vi "Digital Gain (Pre).vi"(0 "data in":T1[](array[typedef])=[{"I"=0.0, "Q"=0.0, "overflow"=FALSE}, {"I"=0.0, "Q"=0.0, "overflow"=FALSE}], 9 "input valid":bool, 11 "gen in":refnum<class "niUSRP Tx DSP v2 FPGA.lvclass">, 12 "ready for output (T)":bool=TRUE) -> (4 "data out":T1[](array[typedef]), 10 "output valid":bool, 14 "ready for input":bool, 15 "gen out":refnum<class "niUSRP Tx DSP v2 FPGA.lvclass">)   [LabVIEW 2025, in "niUSRP Tx DSP v2 FPGA.lvclass"]
uses:
  niUSRP Tx DSP v2 FPGA.lvclass
  <instrlib>/_niInstr/DSP/v1/Shared/Public/IQ Data.ctl
  <instrlib>/_niInstr/DSP Control/Interface/v1/FPGA/Digital Gain/IQ 18-bit/Digital Gain Interface (IQ 18-bit).lvclass
  <instrlib>/_niInstr/Basic Elements/v1/FPGA/niInstr Basic Elements v1 FPGA.lvlib
  <instrlib>/_niInstr/DSP/v1/Shared/niInstr DSP v1 Shared.lvlib
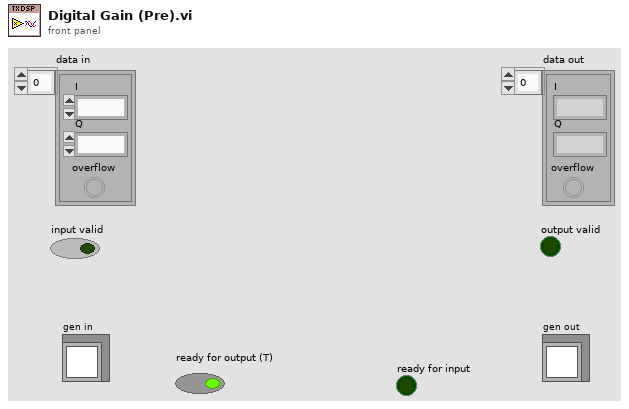
[diagram p1: front panel]
types:
  T1 = typedef "niInstr DSP v1 Shared.lvlib/IQ Data.ctl" = cluster{"I":fxp<+/-,18,1>, "Q":fxp<+/-,18,1>, "overflow":bool}
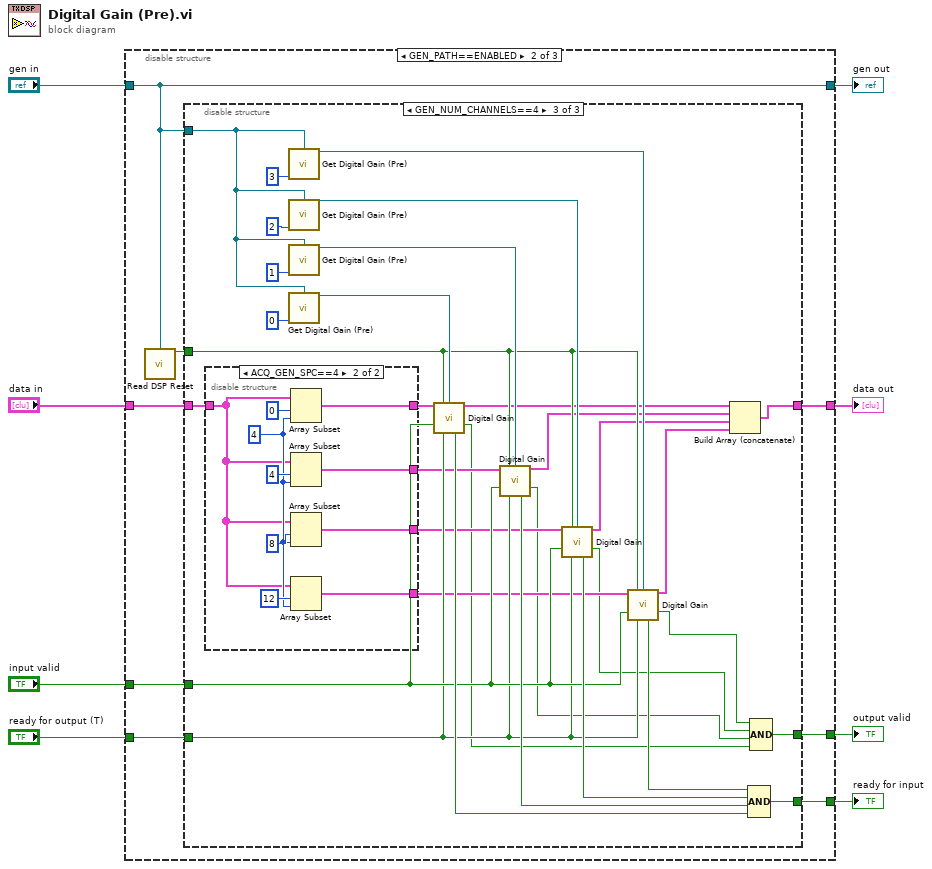
[diagram p0: block diagram]
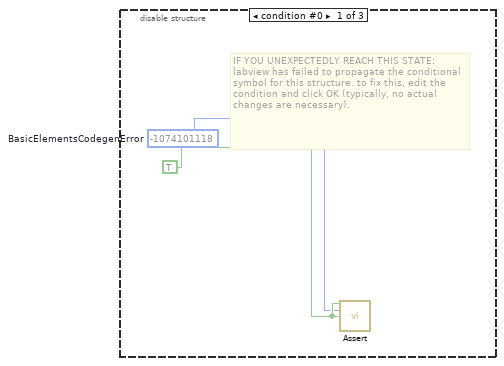
[diagram p2: hidden frame]
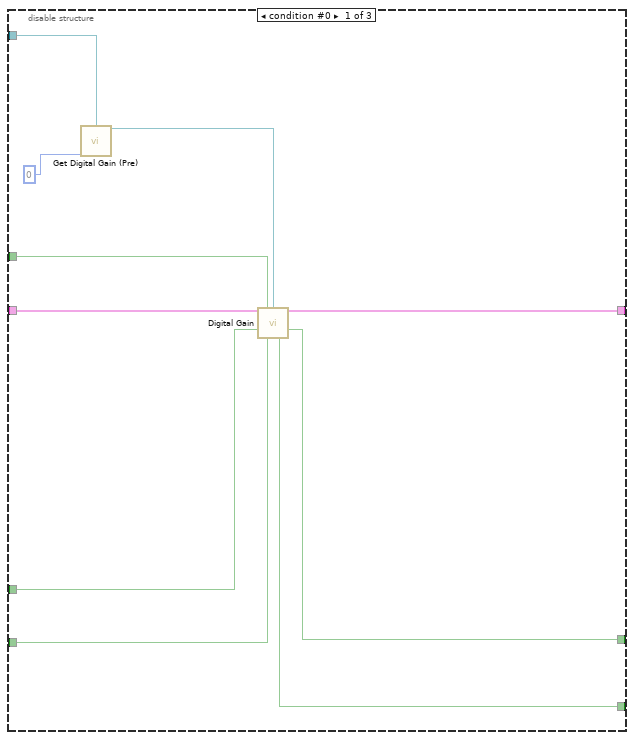
[diagram p3: hidden frame]
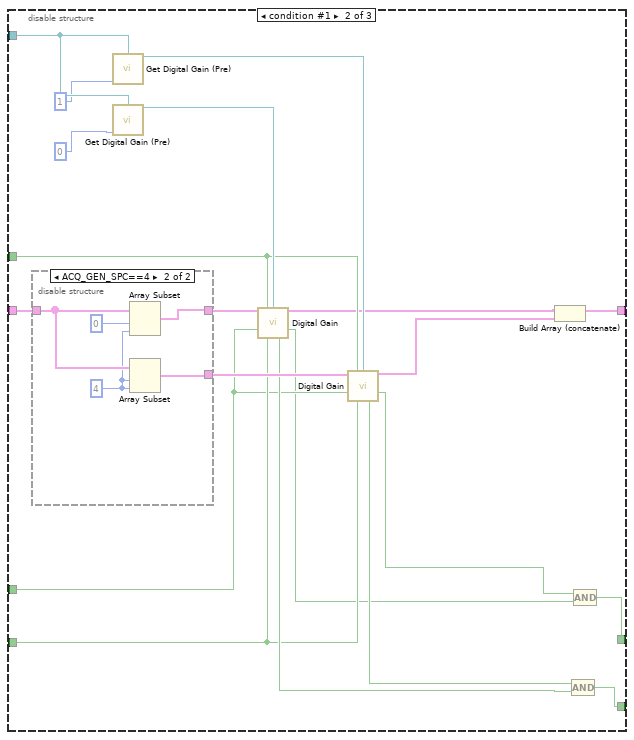
[diagram p4: hidden frame]
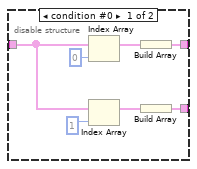
[diagram p5: hidden frame]
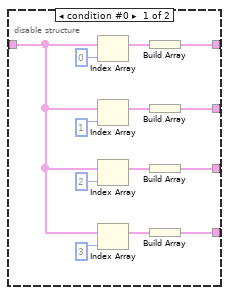
[diagram p6: hidden frame]
diagram:
  n1 = disable-structure shown="GEN_PATH==ENABLED" {
    disable-tunnel: [_ w18 w119] -> w8
    disable-tunnel: "input valid" -> [_ w17 w118]
    disable-tunnel: "ready for output (T)" -> [_ w16 w117]
    disable-tunnel: [_ w15 w118] -> w5
    disable-tunnel: "data in" -> [_ w14 w119]
    disable-tunnel: [_ w13 w117] -> w2
    disable-tunnel: "gen in" -> [_ w11 w116]
    disable-tunnel: [_ w11 w116] -> w1
    frame condition #0 {
      w10 = TRUE ("assert")
      w9 = -1074101118  # BasicElementsCodegenError
      # "IF YOU UNEXPECTEDLY REACH THIS STATE:\nlabview has failed to propagate the conditional symbol for this structure. to fix this, edit the condition and click OK (typically, no actual changes are necessary)."
      n2 = call <instrlib>:"Assert.vi"("assert"=w10, "error code"=w9, "enable show error"=w10) -> ()  [unwired: 13 in]
    }
    frame condition #1 (active) {
      n3 = call-dynamic "Read DSP Reset.vi"("gen"=w11) -> ("dsp reset"=w12:bool)  [unwired: 14 in]
      n4 = disable-structure shown="GEN_NUM_CHANNELS==4" {
        disable-tunnel: [w28 w42 w92] -> w18
        disable-tunnel: w17 -> [w27 w36 w75]
        disable-tunnel: w16 -> [w26 w37 w74]
        disable-tunnel: [w25 w41 w91] -> w15
        disable-tunnel: w14 -> [w24 w46 w73]
        disable-tunnel: [w23 w39 w89] -> w13
        disable-tunnel: w12 -> [w22 w33 w76]
        disable-tunnel: w11 -> [w20 w47 w83]
        frame condition #0 {
          n5 = call-dynamic "Get Digital Gain (Pre).vi"("gen"=w20, "ch"=u8 0) -> ("digital gain"=w21:refnum<class "Digital Gain Interface (IQ 18-bit).lvclass">)  [unwired: 13 in]
          n6 = call-dynamic "Digital Gain.vi"("data in"=w24, "reset"=w22, "digital gain"=w21, "input valid"=w27, "ready for output (T)"=w26) -> ("data out"=w28:T1[], "output valid"=w25:bool, "ready for input"=w23:bool)  [unwired: 7 in, 1 out]
        }
        frame condition #1 {
          n7 = disable-structure shown="ACQ_GEN_SPC==4" {
            disable-tunnel: w46 -> [w51 w58]
            disable-tunnel: [w50 w59] -> w45
            disable-tunnel: [w49 w57] -> w44
            frame condition #0 {
              n8 = Index Array(array=w51, index=0) -> (element=w55:T1)
              n9 = Index Array(array=w51, index=1) -> (element=w53:T1)
              n10 = Build Array(w55) -> (w50:T1[])
              n11 = Build Array(w53) -> (w49:T1[])
            }
            frame condition #1 (active) {
              w56 = 4 ("length")
              n12 = Array Subset(array=w58, index=0, length=w56) -> (w59:T1[])
              n13 = Array Subset(array=w58, index=w56, length=w56) -> (w57:T1[])
            }
          }
          n14 = call-dynamic "Get Digital Gain (Pre).vi"("gen"=w47, "ch"=u8 1) -> ("digital gain"=w43:refnum<class "Digital Gain Interface (IQ 18-bit).lvclass">)  [unwired: 13 in]
          n15 = call-dynamic "Get Digital Gain (Pre).vi"("gen"=w47, "ch"=u8 0) -> ("digital gain"=w48:refnum<class "Digital Gain Interface (IQ 18-bit).lvclass">)  [unwired: 13 in]
          n16 = call-dynamic "Digital Gain.vi"("data in"=w45, "reset"=w33, "digital gain"=w48, "input valid"=w36, "ready for output (T)"=w37) -> ("data out"=w32:T1[], "output valid"=w29:bool, "ready for input"=w40:bool)  [unwired: 7 in, 1 out]
          n17 = call-dynamic "Digital Gain.vi"("data in"=w44, "reset"=w33, "digital gain"=w43, "input valid"=w36, "ready for output (T)"=w37) -> ("data out"=w31:T1[], "output valid"=w30:bool, "ready for input"=w38:bool)  [unwired: 7 in, 1 out]
          n18 = Build Array (concatenate)(w32, w31) -> (w42:T1[])
          n19 = Compound Arithmetic op=AND(w38, w40) -> (w39:bool)
          n20 = Compound Arithmetic op=AND(w30, w29) -> (w41:bool)
        }
        frame condition #2 (active) {
          n21 = disable-structure shown="ACQ_GEN_SPC==4" {
            disable-tunnel: [w101 w109] -> w72
            disable-tunnel: [w100 w108] -> w71
            disable-tunnel: [w99 w107] -> w70
            disable-tunnel: w73 -> [w94 w110]
            disable-tunnel: [w93 w106] -> w69
            frame condition #0 {
              n22 = Index Array(array=w94, index=0) -> (element=w105:T1)
              n23 = Index Array(array=w94, index=1) -> (element=w103:T1)
              n24 = Index Array(array=w94, index=2) -> (element=w95:T1)
              n25 = Index Array(array=w94, index=3) -> (element=w97:T1)
              n26 = Build Array(w105) -> (w101:T1[])
              n27 = Build Array(w103) -> (w100:T1[])
              n28 = Build Array(w95) -> (w99:T1[])
              n29 = Build Array(w97) -> (w93:T1[])
            }
            frame condition #1 (active) {
              w111 = 4 ("length")
              n30 = Array Subset(array=w110, index=0, length=w111) -> (w109:T1[])
              n31 = Array Subset(array=w110, index=4, length=w111) -> (w108:T1[])
              n32 = Array Subset(array=w110, index=8, length=w111) -> (w107:T1[])
              n33 = Array Subset(array=w110, index=12, length=w111) -> (w106:T1[])
            }
          }
          n34 = call-dynamic "Get Digital Gain (Pre).vi"("gen"=w83, "ch"=u8 3) -> ("digital gain"=w77:refnum<class "Digital Gain Interface (IQ 18-bit).lvclass">)  [unwired: 13 in]
          n35 = call-dynamic "Get Digital Gain (Pre).vi"("gen"=w83, "ch"=u8 2) -> ("digital gain"=w78:refnum<class "Digital Gain Interface (IQ 18-bit).lvclass">)  [unwired: 13 in]
          n36 = call-dynamic "Get Digital Gain (Pre).vi"("gen"=w83, "ch"=u8 1) -> ("digital gain"=w81:refnum<class "Digital Gain Interface (IQ 18-bit).lvclass">)  [unwired: 13 in]
          n37 = call-dynamic "Get Digital Gain (Pre).vi"("gen"=w83, "ch"=u8 0) -> ("digital gain"=w82:refnum<class "Digital Gain Interface (IQ 18-bit).lvclass">)  [unwired: 13 in]
          n38 = call-dynamic "Digital Gain.vi"("data in"=w72, "reset"=w76, "digital gain"=w82, "input valid"=w75, "ready for output (T)"=w74) -> ("data out"=w68:T1[], "output valid"=w61:bool, "ready for input"=w90:bool)  [unwired: 7 in, 1 out]
          n39 = call-dynamic "Digital Gain.vi"("data in"=w71, "reset"=w76, "digital gain"=w81, "input valid"=w75, "ready for output (T)"=w74) -> ("data out"=w67:T1[], "output valid"=w62:bool, "ready for input"=w88:bool)  [unwired: 7 in, 1 out]
          n40 = call-dynamic "Digital Gain.vi"("data in"=w70, "reset"=w76, "digital gain"=w78, "input valid"=w75, "ready for output (T)"=w74) -> ("data out"=w66:T1[], "output valid"=w63:bool, "ready for input"=w80:bool)  [unwired: 7 in, 1 out]
          n41 = call-dynamic "Digital Gain.vi"("data in"=w69, "reset"=w76, "digital gain"=w77, "input valid"=w75, "ready for output (T)"=w74) -> ("data out"=w65:T1[], "output valid"=w64:bool, "ready for input"=w79:bool)  [unwired: 7 in, 1 out]
          n42 = Build Array (concatenate)(w68, w67, w66, w65) -> (w92:T1[])
          n43 = Compound Arithmetic op=AND(w79, w80, w88, w90) -> (w89:bool)
          n44 = Compound Arithmetic op=AND(w64, w63, w62, w61) -> (w91:bool)
        }
      }
    }
    frame condition #2 {
    }
  }
  "data out" <- w8
  "output valid" <- w5
  "ready for input" <- w2
  "gen out" <- w1
